vi "Add Component Configuration.vi"(7 "component name":string, 8 "error in (no error)":errorcluster, 10 "Configuration":refnum<class "Configuration.lvclass">, 11 "component settings in":T1[](array[typedef])) -> (0 "error out":errorcluster, 1 "no settings?":bool, 3 "component settings out":T1[](array[typedef]))   [LabVIEW 2019, in "DSF Core.lvlib"]
uses:
  DSF Core.lvlib
  Typedefs/DSF Settings Info.ctl
  Classes/Configuration/Configuration.lvclass
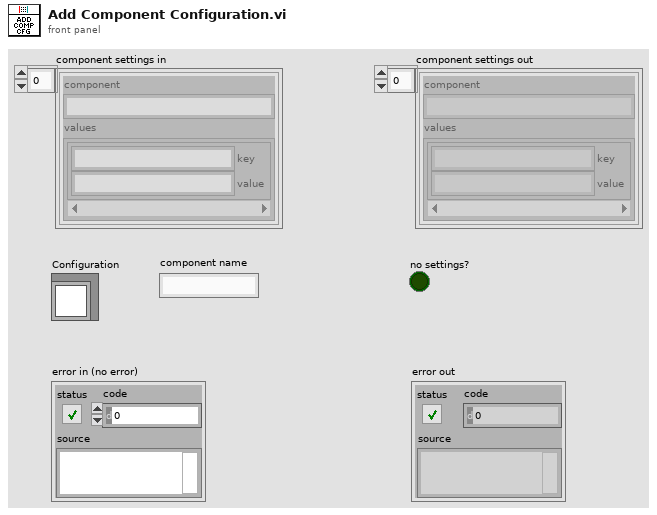
[diagram p1: front panel]
types:
  T1 = typedef "DSF Core.lvlib/DSF Settings Info.ctl" = cluster{"component":string, "values":cluster{"key":string, "value":string}[]}
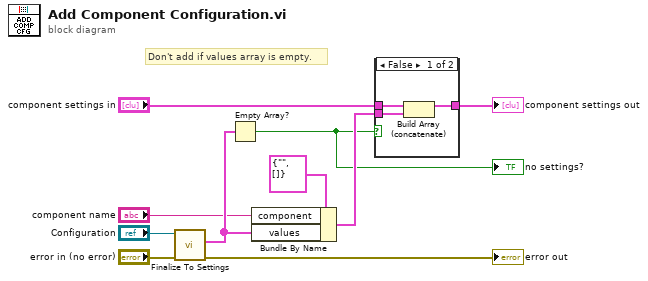
[diagram p0: block diagram]
diagram:
  # "Don't add if values array is empty."
  n1 = call-dynamic "Finalize To Settings.vi"("error in (no error)"="error in (no error)", "Configuration in"="Configuration") -> ("error out"=→"error out":errorcluster, "settings"=w5:cluster{"key":string, "value":string}[])  [unwired: 7 in, 1 out]
  n2 = Empty Array?(array=w5) -> (empty?=w2:bool)
  "no settings?" <- w2
  n3 = Bundle By Name(cluster=T1 {"component"="", "values"=[]} ("component settings out"), "component"="component name", "values"=w5) -> (w4:T1)
  n4 = case shown="False" w2 {
    tunnel: "component settings in" -> [w13 w14]
    tunnel: w4 -> [w12 _]
    tunnel: [w11 w14] -> w3
    frame False {
      n5 = Build Array (concatenate)(w13, w12) -> (w11:T1[])
    }
    frame True {
    }
  }
  "component settings out" <- w3
